vi "CRC16.vi"(4 "string":string="01040FA10008") -> (0 "CRCLo（十进制）":u8=163, 1 "string&CRC":string="01040FA10008A33A", 2 "CRCHi(十进制)":u8=58)   [LabVIEW 2014]
panel:
  out "length":i32=6
  # "字符串转十六进制"
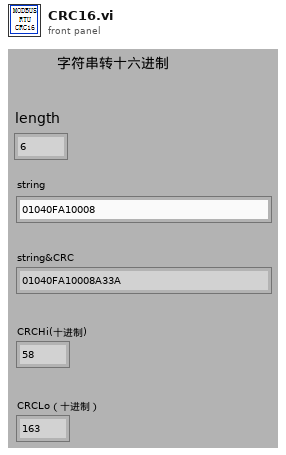
[diagram p1: front panel]
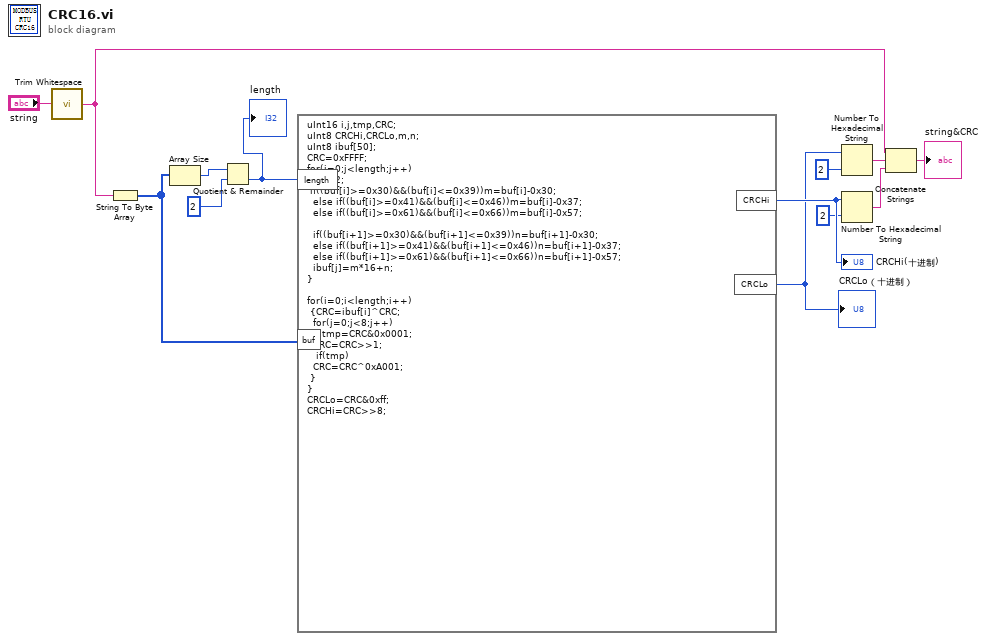
[diagram p0: block diagram]
diagram:
  n1 = call <vilib>:"Trim Whitespace.vi"("string"="string") -> ("trimmed string"=w1:string)  [unwired: 1 in]
  n2 = String To Byte Array ("字符串至字节数组转换")(string=w1) -> (unsigned byte array=w8:u8[])
  n3 = Array Size(array=w8) -> (size(s)=w7:i32)
  n4 = Quotient & Remainder(x=w7, y=2) -> (floor(x/y)=w5:i32)  [unwired: 1 out]
  "length" <- w5
  n5 = formula code="uInt16 i,j,tmp,CRC;\nuInt8 CRCHi,CRCLo,m,n;\nuInt8 ibuf[50];\nCRC=0xFFFF; \nfor(j=0;j<length;j++)\n{ i=j*2;\n if((buf[i]>=0x30)&&(buf[i]<=0x39))m=buf[i]-0x30;\n  else if((buf[i]>=0x41)&&(buf[i]<=0x46))m=buf[i]-0x37;\n  else if((buf[i]>=0x61)&&(buf[i]<=0x66))m=buf[i]-0x57;\n\n  if((buf[i+1]>=0x30)&&(buf[i+1]<=0x39))n=buf[i+1]-0x30;\n  else if((buf[i+1]>=0x41)&&(buf[i+1]<=0x46))n=buf[i+1]-0x37;\n  else if((buf[i+1]>=0x61)&&(buf[i+1]<=0x66))n=buf[i+1]-0x57;\n  ibuf[j]=m*16+n;\n}\n\nfor(i=0;i<length;i++)\n {CRC=ibuf[i]^CRC;\n  for(j=0;j<8;j++)\n   {tmp=CRC&0x0001;\n  CRC=CRC>>1;\n   if(tmp)\n  CRC=CRC^0xA001;\n }\n}\nCRCLo=CRC&0xff;\nCRCHi=CRC>>8;"("buf"=w8, "length"=w5) -> ("CRCHi"=w13:u8, "CRCLo"=w12:u8)
  "CRCHi(十进制)" <- w13
  "CRCLo（十进制）" <- w12
  n6 = Number To Hexadecimal String(1:2, 2:w12) -> (0:w10:string)
  n7 = Number To Hexadecimal String(1:2, 2:w13) -> (0:w9:string)
  n8 = Concatenate Strings(w1, w10, w9) -> (→"string&CRC":string)
